vi "模板.vi"(9 "产品规格":cluster{"产品长度（周长）（mm）":dbl, "产品宽度（母线长）（mm）":dbl}, 10 "临界面积百分比值":dbl, 11 "临界Z值":i32) -> (3 "检测结果":string[][](table))   [LabVIEW 2018]
panel:
  out "原图所在路径":path
  out "结果保存的数据库所在路径":path
  in  "stop 2":bool caption="停止"
  in  "stop":bool caption="停止"
  out "模型预测进度（请等待2-3分钟）":u8(slide) scale=0.0..1000.0
  out "模型所在路径":path
  out "预测图片保存路径":path
  in  "选项卡控件":enum32{"原图", "预测结果"}(tab)
  out "原图":T1(plugin-control)
  out "预测结果图":T1(plugin-control)
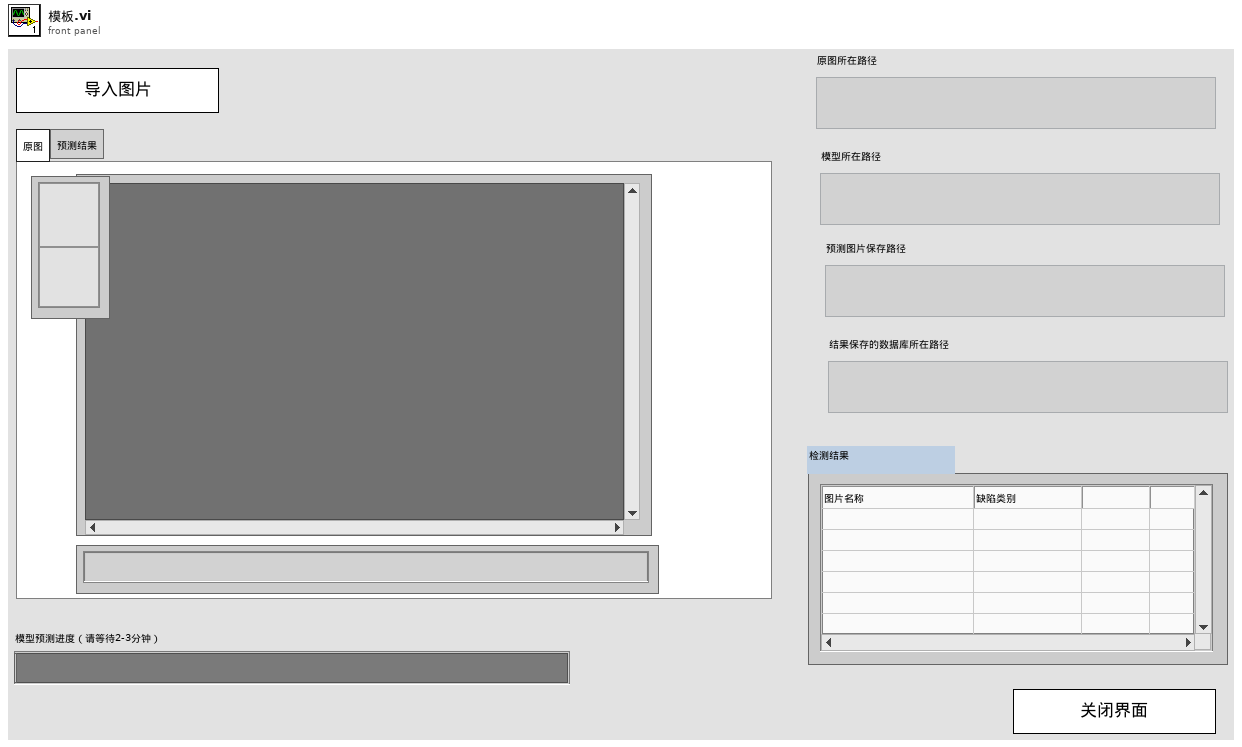
[diagram p1: front panel]
types:
  T1 = typedef "IMAQ Image.ctl" = refnum<image>
  T2 = typedef "Image Type" = u32
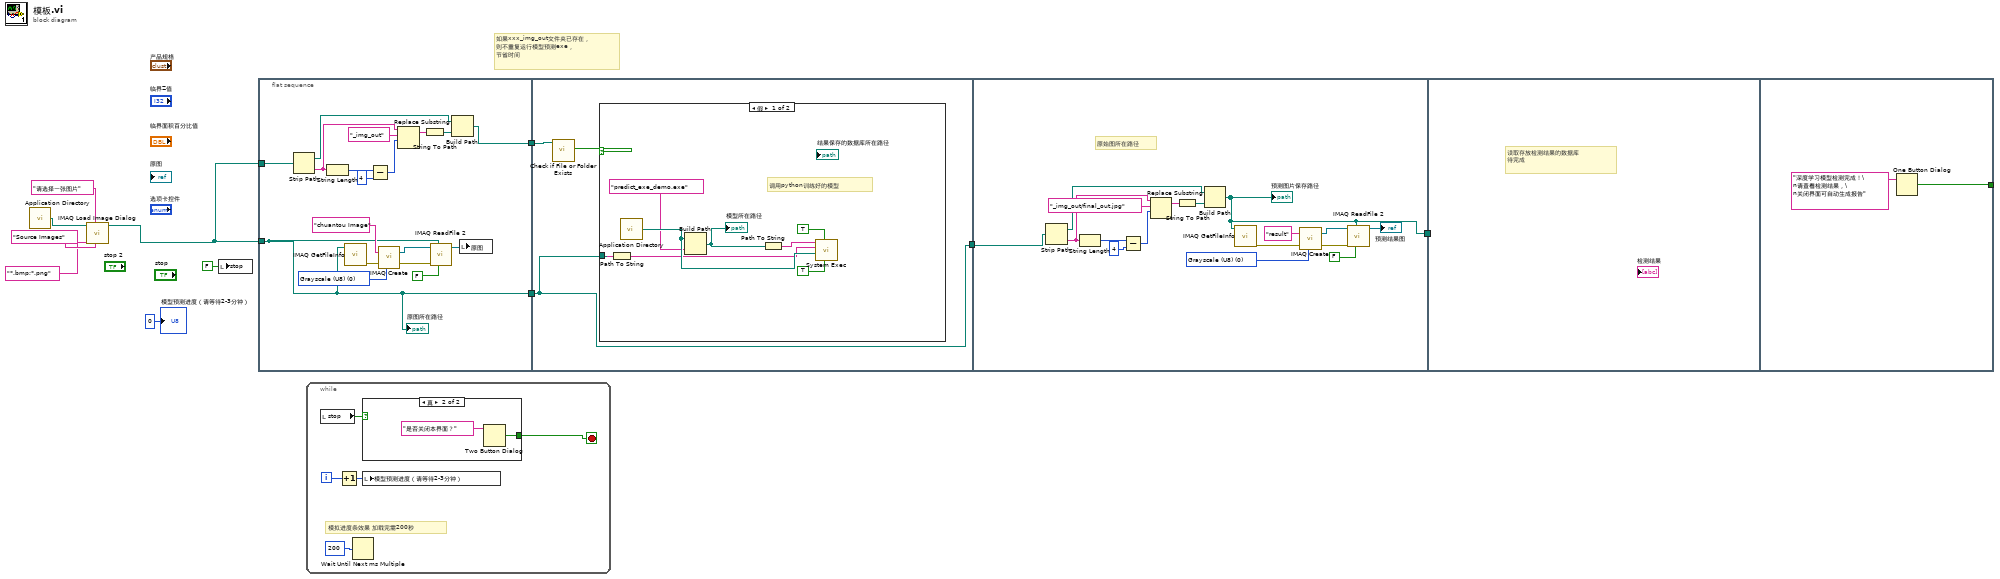
[diagram p0: block diagram]
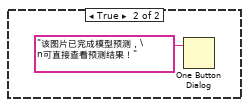
[diagram p2: hidden frame]
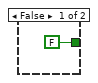
[diagram p3: hidden frame]
diagram:
  # "如果xxx_img_out文件夹已存在，\n则不重复运行模型预测exe，\n节省时间"
  n1 = call <vilib>:"Application Directory.vi"() -> ("Application Directory"=w1:path)
  n2 = call "IMAQ Load Image Dialog"("Pattern Label"="Source Images", "Prompt"="请选择一张图片" ("prompt"), "Pattern"="*.bmp;*.png", "Start Path"=w1) -> ("Path"=w3:path)  [unwired: 5 in, 2 out]
  n3 = local write "stop"(FALSE ("stop")) -> ()
  n4 = flat-sequence {
    tunnel: [w12] -> w10
    tunnel: w3 -> [w12]
    tunnel: w3 -> [w14]
    tunnel: [w13] -> w7
    tunnel: w10 -> [w30]
    tunnel: w7 -> [w32]
    tunnel: [w30] -> w2
    tunnel: [w43] -> w9
    tunnel: w2 -> [w42]
    tunnel: w9 -> [_]
    tunnel: [w59] -> _
    frame #0 {
      w24 = T2 0 items=["Grayscale (U8)", "Grayscale (I16)", "Grayscale (SGL)", "Complex (CSG)", "RGB (U32)", "HSL (U32)", "RGB (U64)", "Grayscale (U16)"] ("Image Type")
      n5 = Strip Path(path=w14) -> (stripped path=w21:path, name=w22:string)
      n6 = String Length(string=w22) -> (length=w19:i32)
      n7 = call "IMAQ GetFileInfo"("File Path"=w12) -> ("error out"=w27:errorcluster)  [unwired: 4 in, 6 out]
      n8 = Subtract(x=w19, y=4) -> (x-y=w18:i32)
      n9 = call "IMAQ Create"("Image Name"="chuantou Image", "Image Type"=w24, "error in (no error)"=w27) -> ("New Image"=w28:T1, "error out"=w29:errorcluster)  [unwired: 2 in]
      n10 = Replace Substring(3:w18, 4:"_img_out" ("字符串"), 5:w22) -> (1:w20:string)  [unwired: 1 in, 1 out]
      n11 = String To Path(string=w20) -> (path=w17:path)
      n12 = call "IMAQ ReadFile 2"("Use File Path Image Type"=FALSE, "File Path"=w12, "error in (no error)"=w29, "Image"=w28) -> ("Image Out"=w26:T1)  [unwired: 3 in, 4 out]
      n13 = Build Path(base path=w21, name or relative path=w17) -> (appended path=w13:path)
      n14 = local write "原图"(w26) -> ()
      "原图所在路径" <- w12
    }
    frame #1 {
      n15 = call <vilib>:"Check if File or Folder Exists.vi"("path"=w32) -> ("file or folder exists?"=w31:bool)  [unwired: 8 in, 2 out]
      n16 = case shown="假" w31 {
        tunnel: w30 -> [w33 _]
        frame False {
          # "调用python训练好的模型"
          n17 = Path To String(path=w33) -> (string=w37:string)
          n18 = call <vilib>:"Application Directory.vi"() -> ("Application Directory"=w38:path)
          n19 = Build Path(base path=w38, name or relative path="predict_exe_demo.exe" ("名称或相对路径")) -> (appended path=w39:path)
          "模型所在路径" <- w39
          n20 = Path To String(path=w39) -> (string=w40:string)
          n21 = call <vilib>:"System Exec.vi"("run minimized? (F)"=TRUE, "wait until completion? (T)"=TRUE, "working directory"=w38, "standard input"=w37, "command line"=w40) -> ()  [unwired: 3 in, 4 out]
        }
        frame True {
          n22 = One Button Dialog(message="该图片已完成模型预测，\n可直接查看预测结果！" ("消息")) -> ()  [unwired: 1 in, 1 out]
        }
      }
    }
    frame #2 {
      w54 = T2 0 items=["Grayscale (U8)", "Grayscale (I16)", "Grayscale (SGL)", "Complex (CSG)", "RGB (U32)", "HSL (U32)", "RGB (U64)", "Grayscale (U16)"] ("Image Type")
      # "原始图所在路径"
      n23 = Strip Path(path=w42) -> (stripped path=w45:path, name=w44:string)
      n24 = String Length(string=w44) -> (length=w49:i32)
      n25 = Subtract(x=w49, y=4) -> (x-y=w50:i32)
      n26 = Replace Substring(3:w50, 4:"_img_out/final_out.jpg" ("字符串"), 5:w44) -> (1:w48:string)  [unwired: 1 in, 1 out]
      n27 = String To Path(string=w48) -> (path=w51:path)
      n28 = Build Path(base path=w45, name or relative path=w51) -> (appended path=w43:path)
      "预测图片保存路径" <- w43
      n29 = call "IMAQ GetFileInfo"("File Path"=w43) -> ("error out"=w56:errorcluster)  [unwired: 4 in, 6 out]
      n30 = call "IMAQ Create"("Image Name"="result", "Image Type"=w54, "error in (no error)"=w56) -> ("New Image"=w57:T1, "error out"=w58:errorcluster)  [unwired: 2 in]
      n31 = call "IMAQ ReadFile 2"("Use File Path Image Type"=FALSE, "File Path"=w43, "error in (no error)"=w58, "Image"=w57) -> ("Image Out"=→"预测结果图":T1)  [unwired: 3 in, 4 out]
    }
    frame #3 {
      # "读取存放检测结果的数据库\n待完成"
    }
    frame #4 {
      n32 = One Button Dialog(message="深度学习模型检测完成！\n请查看检测结果，\n关闭界面可自动生成报告" ("消息")) -> (true=w59:bool)  [unwired: 1 in]
    }
  }
  n33 = while {
    i -> [w63]
    stop <- w61 stop-if-true
    # "模拟进度条效果 加载完需200秒"
    n34 = local read "stop"() -> (w64:bool)
    n35 = Increment(x=w63) -> (x+1=w62:i32)
    n36 = Wait Until Next ms Multiple(millisecond multiple=u32 200 ("毫秒倍数")) -> ()  [unwired: 1 out]
    n37 = case shown="真" w64 {
      tunnel: [FALSE ("T button?") w67] -> w61
      frame False {
      }
      frame True {
        n38 = Two Button Dialog(message="是否关闭本界面？" ("消息")) -> (T button?=w67:bool)  [unwired: 2 in]
      }
    }
    n39 = local write "模型预测进度（请等待2-3分钟）"(w62) -> ()
  }
  "模型预测进度（请等待2-3分钟）" <- u8 0 ("模型运行进度")
